vi "WPI_SerialPortSetTimeout.vi"(8 "error in (no error)":errorcluster, 10 "Timeout Value (ms)":u32=5000, 11 "SerialPortRef":T1) -> (0 "error out":errorcluster, 3 "SerialPortRef":T1)   [LabVIEW 2017]
doc: "Specifies the minimum timeout value, in milliseconds, to use when reading data from or writing data to the serial device.\n\nThis software is licensed. Open the labview\\readme\\WPI Robotics Library Open Source License.txt file for more information."
uses:
  <vilib>/Rock Robotics/WPI/SerialPort/WPI_SerialPortRef.ctl
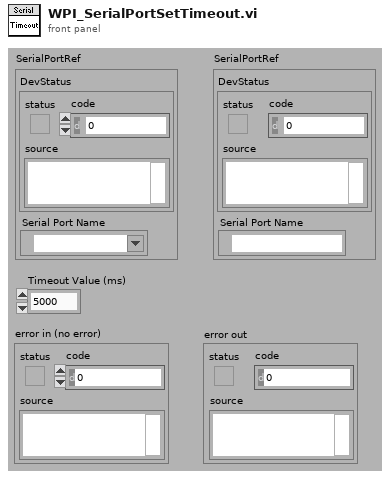
[diagram p1: front panel]
types:
  T1 = typedef "WPI_SerialPortRef.ctl" = cluster{"DevStatus":errorcluster, "Serial Port Name":refnum<visa-resource-name>}
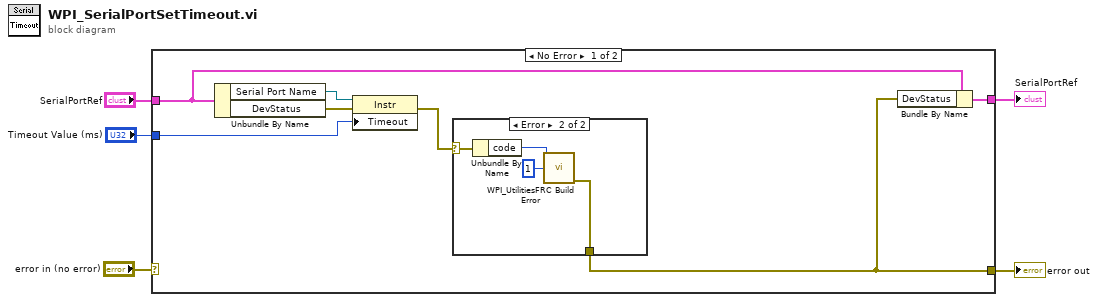
[diagram p0: block diagram]
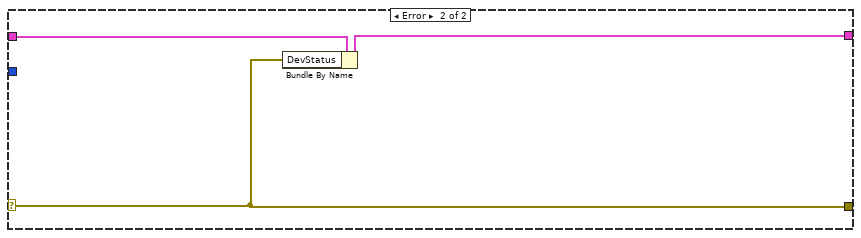
[diagram p3: hidden frame]
diagram:
  n1 = case shown="No Error" "error in (no error)" {
    selector: "error in (no error)" -> [_ w18]
    tunnel: "SerialPortRef" -> [w9 w20]
    tunnel: "Timeout Value (ms)" -> [w12 _]
    tunnel: [w8 w19] -> w4
    tunnel: [w6 w18] -> w2
    frame No Error {
      n2 = Unbundle By Name(w9) -> ("Serial Port Name"=w11:refnum<visa-resource-name>, "DevStatus"=w10:errorcluster)
      n3 = property class="Instr"(reference=w11, error in=w10, "Timeout"=w12) -> (error out=w7:errorcluster)  [unwired: 1 in]
      n4 = case shown="Error" w7 {
        selector: w7 -> [w13 w15]
        tunnel: [w13 w14] -> w6
        frame No Error {
        }
        frame Error {
          n5 = Unbundle By Name(w15) -> ("code"=w17:i32)
          n6 = call <vilib>:"WPI_UtilitiesFRC Build Error.vi"("error code"=w17, "chain levels to remove (1)"=1) -> ("error out"=w14:errorcluster)  [unwired: 3 in, 10 out]
        }
      }
      n7 = Bundle By Name(cluster=w9, "DevStatus"=w6) -> (w8:T1)
    }
    frame Error {
      n8 = Bundle By Name(cluster=w20, "DevStatus"=w18) -> (w19:T1)
    }
  }
  "error out" <- w2
  "SerialPortRef" <- w4
